vi "Goal Vision.vi"() -> ()   [LabVIEW 2015]
uses:
  <vilib>/Rock Robotics/Network Tables/NT Read Number.vi
panel:
  out "Angle":dbl
  in  "X axis field of view (deg)":dbl=70.0
  in  "Image width(px)":dbl=640.0
  out "Distance (in)":dbl
  in  "Y axis field of view (deg)":dbl=51.0
  in  "Image height (px)":dbl=480.0
  in  "Camera Angle (deg)":dbl=30.0
  in  "Camera Height (in)":dbl=18.0
  in  "Target Height (in)":dbl=72.0
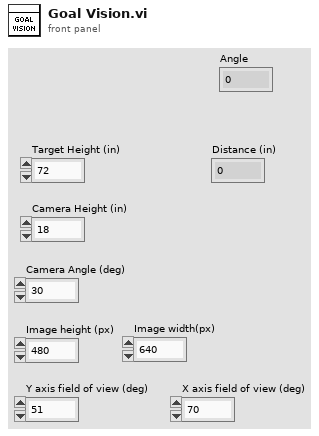
[diagram p1: front panel]
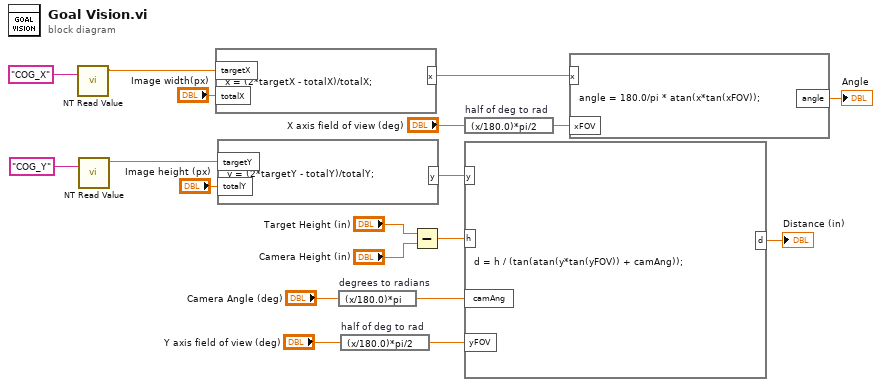
[diagram p0: block diagram]
diagram:
  n1 = call-poly <vilib>:"NT Read Value.vi"("Name"="COG_X") -> ("Numeric"=w5:dbl)  [unwired: 9 in, 1 out]
  n2 = call-poly <vilib>:"NT Read Value.vi"("Name"="COG_Y") -> ("Numeric"=w7:dbl)  [unwired: 9 in, 1 out]
  n3 = formula code="x = (2*targetX - totalX)/totalX;"("targetX"=w5, "totalX"="Image width(px)") -> ("x"=w2:dbl)
  n4 = formula code="y = (2*targetY - totalY)/totalY;"("targetY"=w7, "totalY"="Image height (px)") -> ("y"=w9:dbl)
  n5 = expression code="(x/180.0)*pi" "degrees to radians"("Camera Angle (deg)") -> (w11:dbl)
  n6 = expression code="(x/180.0)*pi/2" "half of deg to rad"("Y axis field of view (deg)") -> (w12:dbl)
  n7 = Subtract(x="Target Height (in)", y="Camera Height (in)") -> (x-y=w10:dbl)
  n8 = expression code="(x/180.0)*pi/2" "half of deg to rad"("X axis field of view (deg)") -> (w3:dbl)
  n9 = formula code="d = h / (tan(atan(y*tan(yFOV)) + camAng));"("y"=w9, "h"=w10, "camAng"=w11, "yFOV"=w12) -> ("d"=→"Distance (in)":dbl)
  n10 = formula code="angle = 180.0/pi * atan(x*tan(xFOV));"("xFOV"=w3, "x"=w2) -> ("angle"=→"Angle":dbl)
